vi "FT10_FPGA_7854R_Main 3.vi"(0 "Conn1/DIO_0_7 In":bool[](array[boolean])=[FALSE, FALSE, FALSE, FALSE, FALSE, FALSE, FALSE, FALSE], 1 "Conn1/DIO_8_15 In":bool[](array[boolean])=[FALSE, FALSE, FALSE, FALSE, FALSE, FALSE, FALSE, FALSE], 2 "Conn1/DIO_16_23 In":bool[](array[boolean])=[FALSE, FALSE, FALSE, FALSE, FALSE, FALSE, FALSE, FALSE], 3 "Conn2/DIO_0_7 In":bool[](array[boolean])=[FALSE, FALSE, FALSE, FALSE, FALSE, FALSE, FALSE, FALSE], 4 "Conn2/DIO_8_15 In":bool[](array[boolean])=[FALSE, FALSE, FALSE, FALSE, FALSE, FALSE, FALSE, FALSE], 5 "Conn2/DIO_16_23 In":bool[](array[boolean])=[FALSE, FALSE, FALSE, FALSE, FALSE, FALSE, FALSE, FALSE], 6 "Conn1 - 75kHz":bool, 7 "Conn2 - 75kHz":bool, 8 "Conn1 - uSec On":u16 caption="uSec On", 9 "Conn2 - uSec On":u16 caption="uSec On", 10 "Conn1 - uSec Off":u16 caption="uSec Off", 11 "Conn2 - uSec Off":u16 caption="uSec Off") -> (14 "Conn1/DIO_0_7 Out":bool[](array[boolean]), 15 "Conn1/DIO_8_15 Out":bool[](array[boolean]), 16 "Conn1/DIO_16_23 Out":bool[](array[boolean]), 17 "Conn2/DIO_0_7 Out":bool[](array[boolean]), 18 "Conn2/DIO_8_15 Out":bool[](array[boolean]), 19 "Conn2/DIO_16_23 Out":bool[](array[boolean]))   [LabVIEW 2024]
uses:
  <vilib>/rvi/Emulation/niFpgaGetClockAttributes.vi
  <vilib>/rvi/Emulation/niFpgaSctlEmulationGetInTimedLoop.vi
  <vilib>/rvi/Emulation/niFpgaEmulationReportErrorSimple.vi
  <vilib>/rvi/eio/common/nirviEmuTemplateMethod_errors.vi
  <vilib>/rvi/Emulation/niFpgaCriticalErrorInLSC.vi
  <vilib>/eio/EIONode/EIONode.xnode
panel:
  # "Inputs"
  # "Outputs"
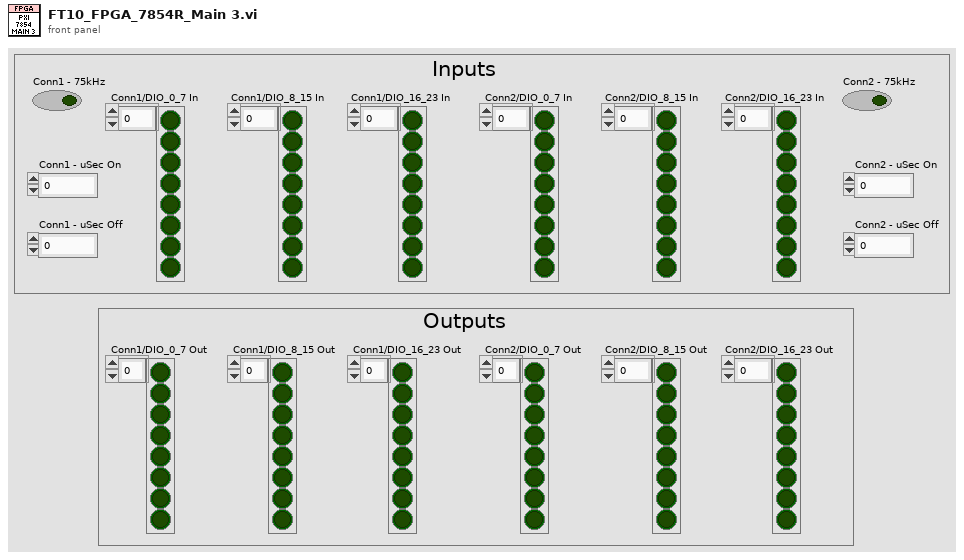
[diagram p1: front panel]
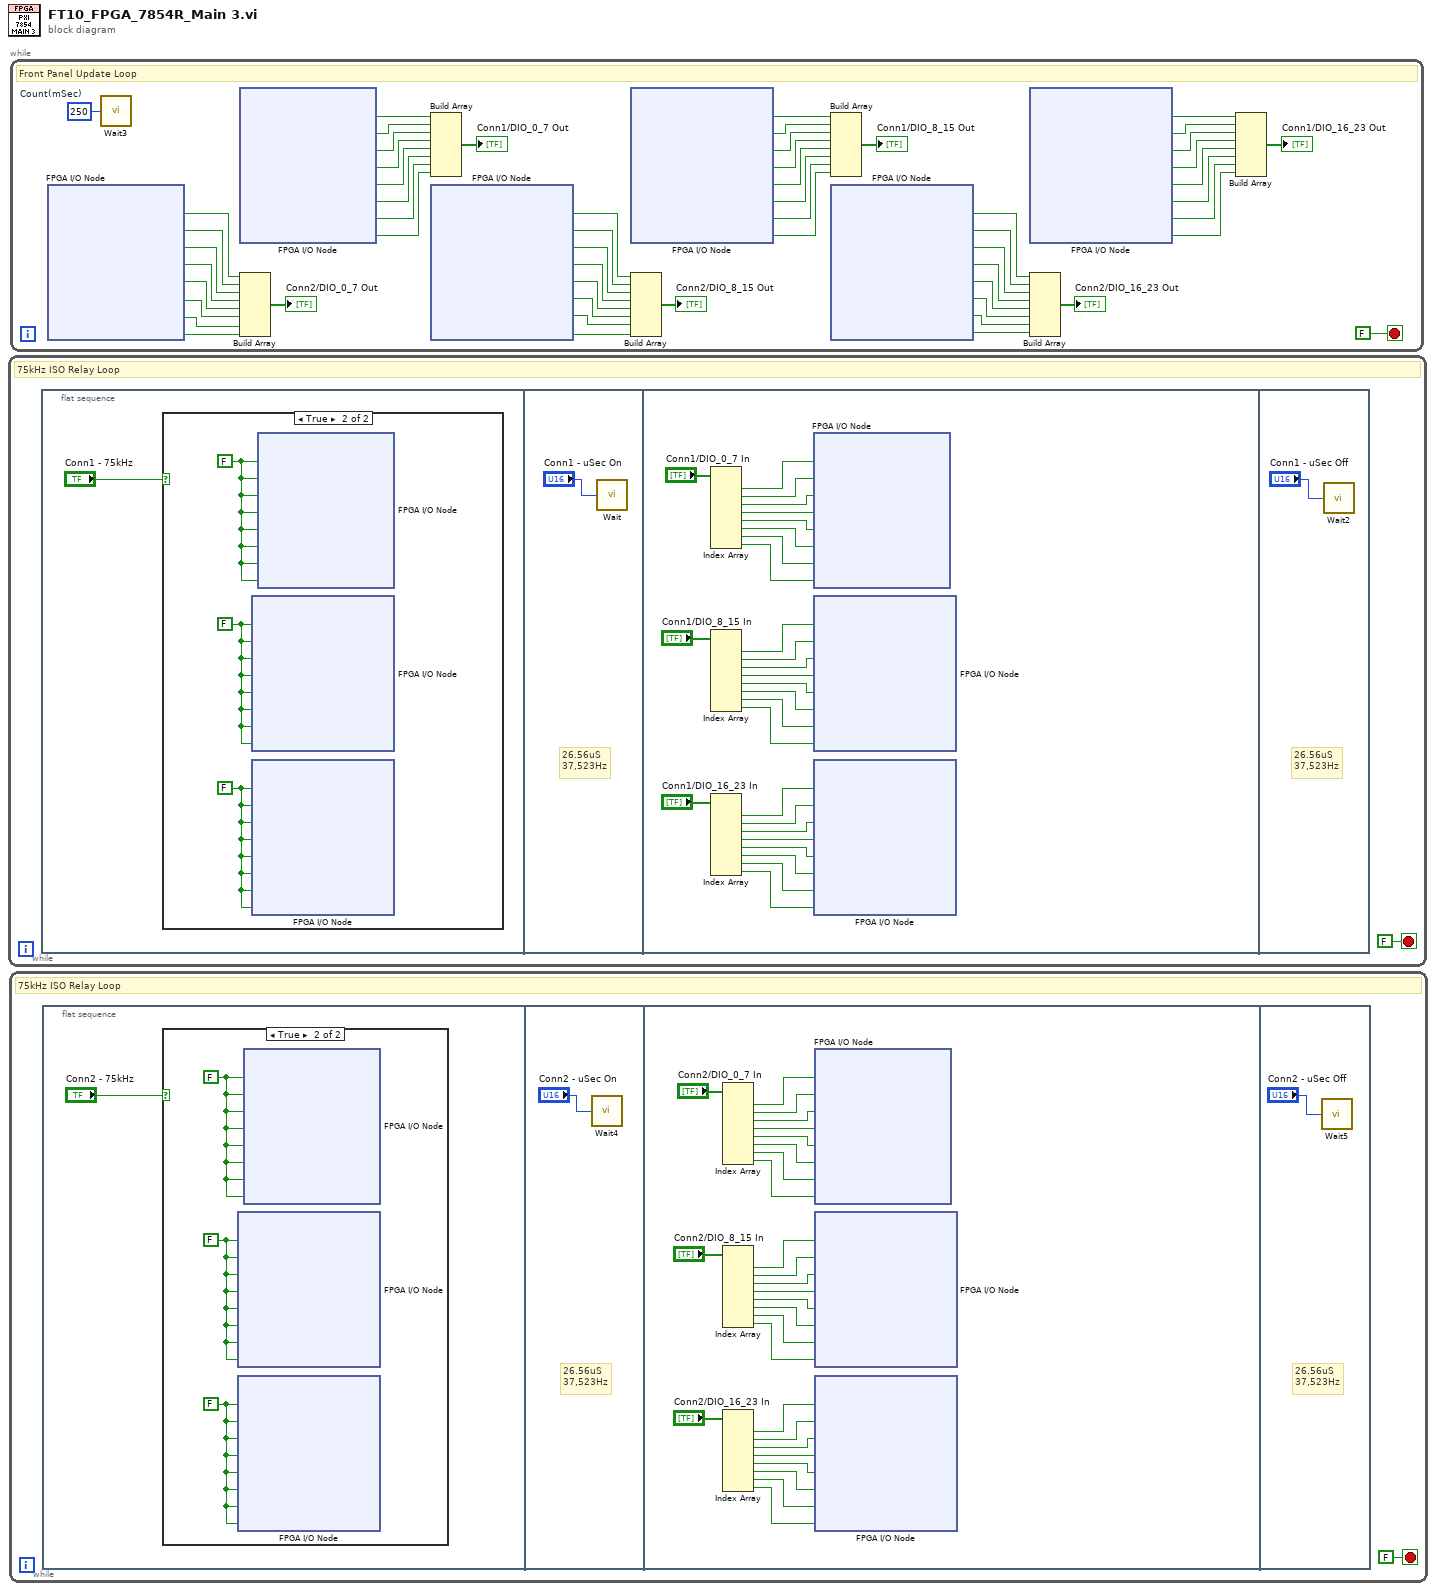
[diagram p0: block diagram]
diagram:
  n1 = while {
    stop <- FALSE stop-if-true
    # "75kHz ISO Relay Loop"
    n2 = flat-sequence {
      frame #0 {
        n3 = case shown="True" "Conn1 - 75kHz" {
          frame False {
          }
          frame True {
            w5 = FALSE ("Connector1/DIO16")
            w4 = FALSE ("Connector1/DIO8")
            w3 = FALSE ("Connector1/DIO0")
            n4 = xnode "FPGA I/O Node"("Connector1/DIO8"=w4, "Connector1/DIO9"=w4, "Connector1/DIO10"=w4, "Connector1/DIO11"=w4, "Connector1/DIO12"=w4, "Connector1/DIO13"=w4, "Connector1/DIO14"=w4, "Connector1/DIO15"=w4) -> ()  [unwired: 8 in, 8 out]
            n5 = xnode "FPGA I/O Node"("Connector1/DIO16"=w5, "Connector1/DIO17"=w5, "Connector1/DIO18"=w5, "Connector1/DIO19"=w5, "Connector1/DIO20"=w5, "Connector1/DIO21"=w5, "Connector1/DIO22"=w5, "Connector1/DIO23"=w5) -> ()  [unwired: 8 in, 8 out]
            n6 = xnode "FPGA I/O Node"("Connector1/DIO0"=w3, "Connector1/DIO1"=w3, "Connector1/DIO2"=w3, "Connector1/DIO3"=w3, "Connector1/DIO4"=w3, "Connector1/DIO5"=w3, "Connector1/DIO6"=w3, "Connector1/DIO7"=w3) -> ()  [unwired: 8 in, 8 out]
          }
        }
      }
      frame #1 {
        # "26.56uS\n37,523Hz"
        n7 = call "Wait"("Count(uSec)"="Conn1 - uSec On") -> ()  [unwired: 1 out]
      }
      frame #2 {
        n8 = Index Array(array="Conn1/DIO_0_7 In") -> (element #1=w20:bool, element #2=w19:bool, element #3=w18:bool, element #4=w17:bool, element #5=w16:bool, element #6=w15:bool, element #7=w14:bool, element #8=w21:bool)  [unwired: 8 in]
        n9 = Index Array(array="Conn1/DIO_8_15 In") -> (element #1=w13:bool, element #2=w12:bool, element #3=w11:bool, element #4=w10:bool, element #5=w7:bool, element #6=w8:bool, element #7=w9:bool, element #8=w22:bool)  [unwired: 8 in]
        n10 = Index Array(array="Conn1/DIO_16_23 In") -> (element #1=w30:bool, element #2=w29:bool, element #3=w28:bool, element #4=w27:bool, element #5=w26:bool, element #6=w25:bool, element #7=w24:bool, element #8=w23:bool)  [unwired: 8 in]
        n11 = xnode "FPGA I/O Node"("Connector1/DIO0"=w20, "Connector1/DIO1"=w19, "Connector1/DIO2"=w18, "Connector1/DIO3"=w17, "Connector1/DIO4"=w16, "Connector1/DIO5"=w15, "Connector1/DIO6"=w14, "Connector1/DIO7"=w21) -> ()  [unwired: 8 in, 8 out]
        n12 = xnode "FPGA I/O Node"("Connector1/DIO8"=w13, "Connector1/DIO9"=w12, "Connector1/DIO10"=w11, "Connector1/DIO11"=w10, "Connector1/DIO12"=w7, "Connector1/DIO13"=w8, "Connector1/DIO14"=w9, "Connector1/DIO15"=w22) -> ()  [unwired: 8 in, 8 out]
        n13 = xnode "FPGA I/O Node"("Connector1/DIO16"=w30, "Connector1/DIO17"=w29, "Connector1/DIO18"=w28, "Connector1/DIO19"=w27, "Connector1/DIO20"=w26, "Connector1/DIO21"=w25, "Connector1/DIO22"=w24, "Connector1/DIO23"=w23) -> ()  [unwired: 8 in, 8 out]
      }
      frame #3 {
        # "26.56uS\n37,523Hz"
        n14 = call "Wait2"("Count(uSec)"="Conn1 - uSec Off") -> ()  [unwired: 1 out]
      }
    }
  }
  n15 = while {
    stop <- FALSE stop-if-true
    # "75kHz ISO Relay Loop"
    n16 = flat-sequence {
      frame #0 {
        n17 = case shown="True" "Conn2 - 75kHz" {
          frame False {
          }
          frame True {
            w37 = FALSE ("Connector2/DIO8")
            w39 = FALSE ("Connector2/DIO8")
            w38 = FALSE ("Connector2/DIO0")
            n18 = xnode "FPGA I/O Node"("Connector2/DIO8"=w39, "Connector2/DIO9"=w39, "Connector2/DIO10"=w39, "Connector2/DIO11"=w39, "Connector2/DIO12"=w39, "Connector2/DIO13"=w39, "Connector2/DIO14"=w39, "Connector2/DIO15"=w39) -> ()  [unwired: 8 in, 8 out]
            n19 = xnode "FPGA I/O Node"("Connector2/DIO16"=w37, "Connector2/DIO17"=w37, "Connector2/DIO18"=w37, "Connector2/DIO19"=w37, "Connector2/DIO20"=w37, "Connector2/DIO21"=w37, "Connector2/DIO22"=w37, "Connector2/DIO23"=w37) -> ()  [unwired: 8 in, 8 out]
            n20 = xnode "FPGA I/O Node"("Connector2/DIO0"=w38, "Connector2/DIO1"=w38, "Connector2/DIO2"=w38, "Connector2/DIO3"=w38, "Connector2/DIO4"=w38, "Connector2/DIO5"=w38, "Connector2/DIO6"=w38, "Connector2/DIO7"=w38) -> ()  [unwired: 8 in, 8 out]
          }
        }
      }
      frame #1 {
        # "26.56uS\n37,523Hz"
        n21 = call "Wait4"("Count(uSec)"="Conn2 - uSec On") -> ()  [unwired: 1 out]
      }
      frame #2 {
        n22 = Index Array(array="Conn2/DIO_0_7 In") -> (element #1=w65:bool, element #2=w64:bool, element #3=w63:bool, element #4=w62:bool, element #5=w61:bool, element #6=w60:bool, element #7=w59:bool, element #8=w58:bool)  [unwired: 8 in]
        n23 = Index Array(array="Conn2/DIO_8_15 In") -> (element #1=w57:bool, element #2=w56:bool, element #3=w55:bool, element #4=w54:bool, element #5=w53:bool, element #6=w52:bool, element #7=w51:bool, element #8=w50:bool)  [unwired: 8 in]
        n24 = Index Array(array="Conn2/DIO_16_23 In") -> (element #1=w48:bool, element #2=w47:bool, element #3=w46:bool, element #4=w45:bool, element #5=w44:bool, element #6=w43:bool, element #7=w42:bool, element #8=w41:bool)  [unwired: 8 in]
        n25 = xnode "FPGA I/O Node"("Connector2/DIO0"=w65, "Connector2/DIO1"=w64, "Connector2/DIO2"=w63, "Connector2/DIO3"=w62, "Connector2/DIO4"=w61, "Connector2/DIO5"=w60, "Connector2/DIO6"=w59, "Connector2/DIO7"=w58) -> ()  [unwired: 8 in, 8 out]
        n26 = xnode "FPGA I/O Node"("Connector2/DIO8"=w57, "Connector2/DIO9"=w56, "Connector2/DIO10"=w55, "Connector2/DIO11"=w54, "Connector2/DIO12"=w53, "Connector2/DIO13"=w52, "Connector2/DIO14"=w51, "Connector2/DIO15"=w50) -> ()  [unwired: 8 in, 8 out]
        n27 = xnode "FPGA I/O Node"("Connector2/DIO16"=w48, "Connector2/DIO17"=w47, "Connector2/DIO18"=w46, "Connector2/DIO19"=w45, "Connector2/DIO20"=w44, "Connector2/DIO21"=w43, "Connector2/DIO22"=w42, "Connector2/DIO23"=w41) -> ()  [unwired: 8 in, 8 out]
      }
      frame #3 {
        # "26.56uS\n37,523Hz"
        n28 = call "Wait5"("Count(uSec)"="Conn2 - uSec Off") -> ()  [unwired: 1 out]
      }
    }
  }
  n29 = while {
    stop <- FALSE stop-if-true
    w123 = u8 250  # Count(mSec)
    # "Front Panel Update Loop"
    n30 = xnode "FPGA I/O Node"() -> ("Connector2/DIO0"=w122:bool, "Connector2/DIO1"=w121:bool, "Connector2/DIO2"=w120:bool, "Connector2/DIO3"=w104:bool, "Connector2/DIO4"=w119:bool, "Connector2/DIO5"=w118:bool, "Connector2/DIO6"=w117:bool, "Connector2/DIO7"=w116:bool)  [unwired: 8 in, 8 out]
    n31 = call "Wait3"("Count(mSec)"=w123) -> ()  [unwired: 1 out]
    n32 = xnode "FPGA I/O Node"() -> ("Connector1/DIO0"=w102:bool, "Connector1/DIO1"=w101:bool, "Connector1/DIO2"=w100:bool, "Connector1/DIO3"=w99:bool, "Connector1/DIO4"=w98:bool, "Connector1/DIO5"=w97:bool, "Connector1/DIO6"=w96:bool, "Connector1/DIO7"=w95:bool)  [unwired: 8 in, 8 out]
    n33 = Build Array(w122, w121, w120, w104, w119, w118, w117, w116) -> (→"Conn2/DIO_0_7 Out":bool[])
    n34 = Build Array(w102, w101, w100, w99, w98, w97, w96, w95) -> (→"Conn1/DIO_0_7 Out":bool[])
    n35 = xnode "FPGA I/O Node"() -> ("Connector2/DIO8"=w114:bool, "Connector2/DIO9"=w113:bool, "Connector2/DIO10"=w112:bool, "Connector2/DIO11"=w94:bool, "Connector2/DIO12"=w93:bool, "Connector2/DIO13"=w92:bool, "Connector2/DIO14"=w91:bool, "Connector2/DIO15"=w111:bool)  [unwired: 8 in, 8 out]
    n36 = xnode "FPGA I/O Node"() -> ("Connector1/DIO8"=w87:bool, "Connector1/DIO9"=w89:bool, "Connector1/DIO10"=w88:bool, "Connector1/DIO11"=w86:bool, "Connector1/DIO12"=w85:bool, "Connector1/DIO13"=w84:bool, "Connector1/DIO14"=w83:bool, "Connector1/DIO15"=w82:bool)  [unwired: 8 in, 8 out]
    n37 = Build Array(w114, w113, w112, w94, w93, w92, w91, w111) -> (→"Conn2/DIO_8_15 Out":bool[])
    n38 = Build Array(w87, w89, w88, w86, w85, w84, w83, w82) -> (→"Conn1/DIO_8_15 Out":bool[])
    n39 = xnode "FPGA I/O Node"() -> ("Connector2/DIO16"=w109:bool, "Connector2/DIO17"=w107:bool, "Connector2/DIO18"=w106:bool, "Connector2/DIO19"=w81:bool, "Connector2/DIO20"=w80:bool, "Connector2/DIO21"=w79:bool, "Connector2/DIO22"=w78:bool, "Connector2/DIO23"=w105:bool)  [unwired: 8 in, 8 out]
    n40 = xnode "FPGA I/O Node"() -> ("Connector1/DIO16"=w76:bool, "Connector1/DIO17"=w75:bool, "Connector1/DIO18"=w74:bool, "Connector1/DIO19"=w73:bool, "Connector1/DIO20"=w72:bool, "Connector1/DIO21"=w71:bool, "Connector1/DIO22"=w70:bool, "Connector1/DIO23"=w69:bool)  [unwired: 8 in, 8 out]
    n41 = Build Array(w109, w107, w106, w81, w80, w79, w78, w105) -> (→"Conn2/DIO_16_23 Out":bool[])
    n42 = Build Array(w76, w75, w74, w73, w72, w71, w70, w69) -> (→"Conn1/DIO_16_23 Out":bool[])
  }
